vi "Lab 4.vi"() -> ()   [LabVIEW 2018]
panel:
  in  "Physical Channels":tag
  out "Waveform Chart":dynamicdata(graph)
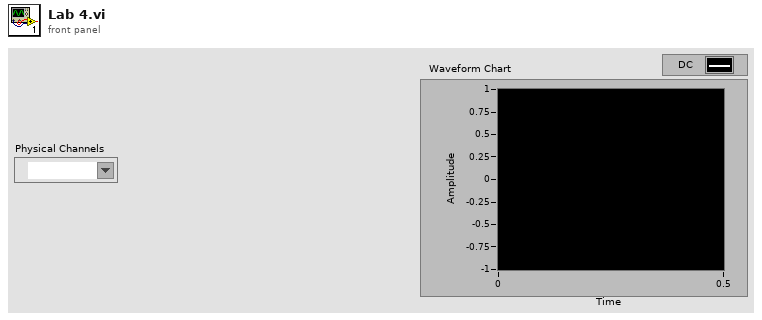
[diagram p1: front panel]
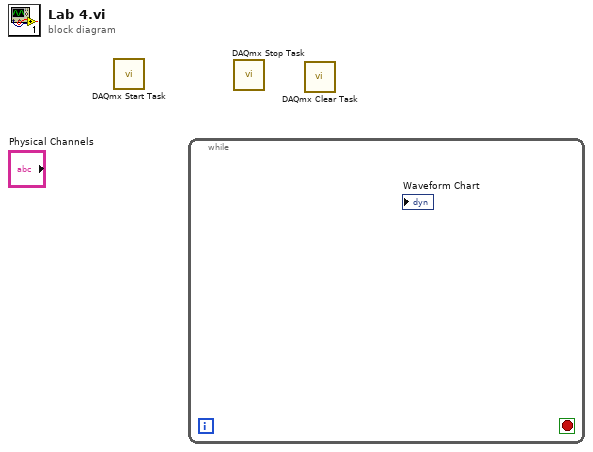
[diagram p0: block diagram]
diagram:
  n1 = call <vilib>:"DAQmx Start Task.vi"() -> ()  [unwired: 14 in, 2 out]
  n2 = while {
    stop <- _ stop-if-true
  }
  n3 = call <vilib>:"DAQmx Stop Task.vi"() -> ()  [unwired: 14 in, 2 out]
  n4 = call <vilib>:"DAQmx Clear Task.vi"() -> ()  [unwired: 15 in, 1 out]
